vi "DMM Measurement Loop.vi"(3 "error in":errorcluster, 4 "DMM Control References Array":T1, 5 "DMM Semaphore":T2) -> (0 "error out":errorcluster)   [LabVIEW 2020]
uses:
  Typedefs/DMM Control Variable References.ctl
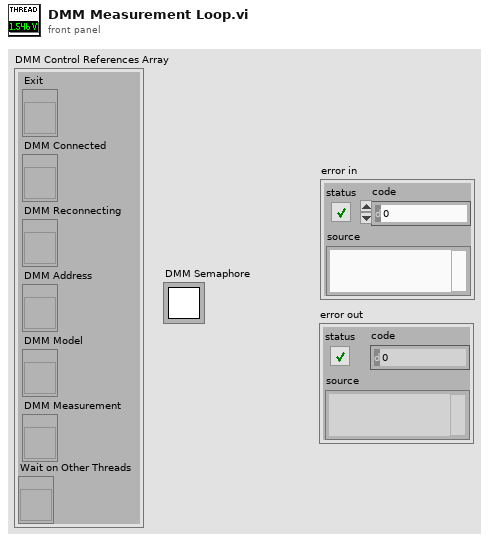
[diagram p1: front panel]
types:
  T1 = typedef "DMM Control Variable References.ctl" = cluster{"Exit":refnum<vi>, "DMM Connected":refnum<vi>, "DMM Reconnecting":refnum<vi>, "DMM Address":refnum<vi>, "DMM Model":refnum<vi>, "DMM Measurement":refnum<vi>, "Wait on Other Threads":refnum<vi>}
  T2 = typedef "Semaphore RefNum" = refnum<k1>
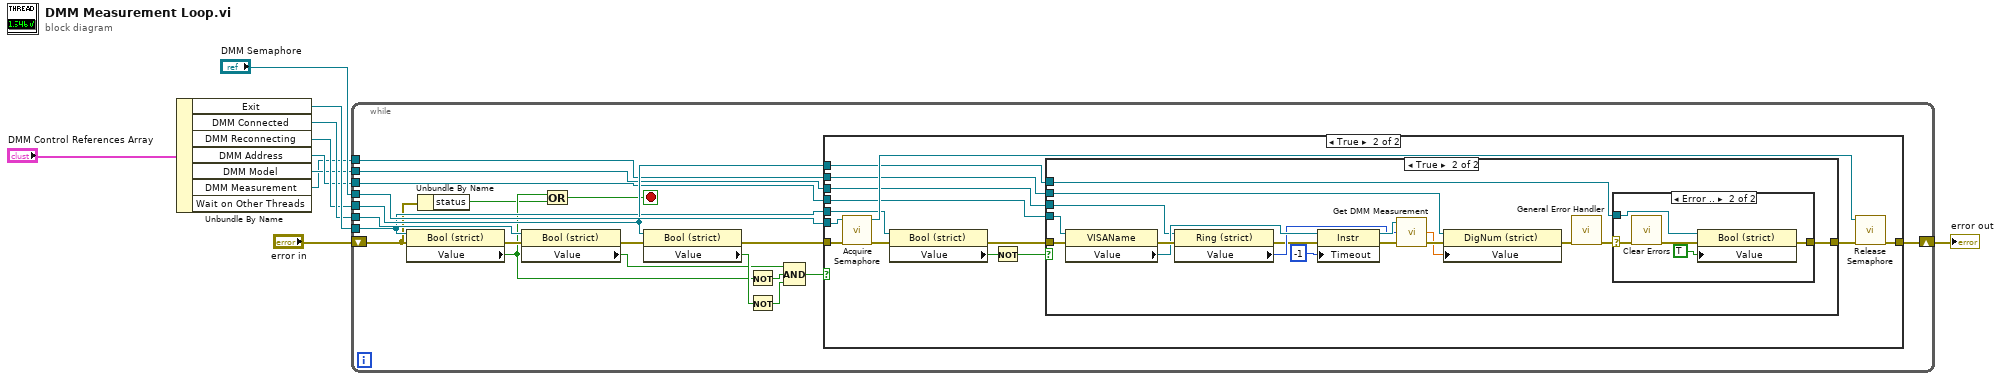
[diagram p0: block diagram]
diagram:
  n1 = Unbundle By Name("DMM Control References Array") -> ("Exit"=w8:refnum<vi>, "DMM Connected"=w7:refnum<vi>, "DMM Reconnecting"=w6:refnum<vi>, "DMM Address"=w5:refnum<vi>, "DMM Model"=w4:refnum<vi>, "DMM Measurement"=w3:refnum<vi>)  [unwired: 1 out]
  n2 = while {
    tunnel: "DMM Semaphore" -> [w30]
    tunnel: w8 -> [w16]
    tunnel: w7 -> [w26]
    tunnel: w6 -> [w20]
    tunnel: w5 -> [w19]
    tunnel: w4 -> [w18]
    tunnel: w3 -> [w17]
    shift-right: [w15] -> w1
    shift-left: "error in" -> [w14]
    stop <- w11 stop-if-true
    n3 = property class="Bool (strict)"(reference=w16, error in=w14) -> (error out=w24:errorcluster, "Value"=w13:bool)  [unwired: 1 out]
    n4 = Unbundle By Name(w14) -> ("status"=w12:bool)
    n5 = property class="Bool (strict)"(reference=w26, error in=w24) -> (error out=w23:errorcluster, "Value"=w21:bool)  [unwired: 1 out]
    n6 = Or(x=w13, y=w12) -> (x .or. y?=w11:bool)
    n7 = property class="Bool (strict)"(reference=w20, error in=w23) -> (error out=w22:errorcluster, "Value"=w25:bool)  [unwired: 1 out]
    n8 = Not(x=w13) -> (.not. x?=w29:bool)
    n9 = Not(x=w25) -> (.not. x?=w28:bool)
    n10 = Compound Arithmetic op=AND(w21, w29, w28) -> (w27:bool)
    n11 = case shown="True" w27 {
      tunnel: w30 -> [_ w45]
      tunnel: w22 -> [w31 w41]
      tunnel: w20 -> [_ w40]
      tunnel: w19 -> [_ w39]
      tunnel: w18 -> [_ w38]
      tunnel: w17 -> [_ w37]
      tunnel: w16 -> [_ w35]
      tunnel: [w31 w32] -> w15
      frame False {
      }
      frame True {
        n12 = call <vilib>:"Acquire Semaphore.vi"("error in (no error)"=w41, "semaphore"=w45) -> ("error out"=w36:errorcluster, "semaphore out"=w43:T2)  [unwired: 3 in, 1 out]
        n13 = property class="Bool (strict)"(reference=w35, error in=w36) -> (error out=w33:errorcluster, "Value"=w34:bool)  [unwired: 1 out]
        n14 = Not(x=w34) -> (.not. x?=w42:bool)
        n15 = case shown="True" w42 {
          tunnel: w33 -> [w46 w57]
          tunnel: [w46 w62] -> w44
          tunnel: w40 -> [_ w58]
          tunnel: w39 -> [_ w55]
          tunnel: w38 -> [_ w53]
          tunnel: w37 -> [_ w50]
          frame False {
          }
          frame True {
            n16 = property class="VISAName"(reference=w55, error in=w57) -> (error out=w56:errorcluster, "Value"=w54:refnum<visa-resource-name>)  [unwired: 1 out]
            n17 = property class="Ring (strict)"(reference=w53, error in=w56) -> (error out=w51:errorcluster, "Value"=w52:u16)  [unwired: 1 out]
            n18 = property class="Instr"(reference=w54, error in=w51, "Timeout"=-1) -> (reference out=w60:refnum<visa-resource-name>, error out=w59:errorcluster)
            n19 = call "Get DMM Measurement.vi"("error in"=w59, "DMM Model"=w52, "DMM Address"=w60) -> ("error out"=w49:errorcluster, "Measurement"=w47:dbl)  [unwired: 1 out]
            n20 = property class="DigNum (strict)"(reference=w50, error in=w49, "Value"=w47) -> (error out=w48:errorcluster)  [unwired: 1 out]
            n21 = call <vilib>:"General Error Handler.vi"("error in (no error)"=w48) -> ("error out"=w63:errorcluster)  [unwired: 10 in, 4 out]
            n22 = case shown="Error .." w63 {
              selector: w63 -> [w64 w69]
              tunnel: [w64 w65] -> w62
              tunnel: w58 -> [_ w68]
              frame No Error {
              }
              frame Error {
                n23 = call <vilib>:"Clear Errors.vi"("error in (no error)"=w69) -> ("error out"=w66:errorcluster)  [unwired: 5 in, 1 out]
                n24 = property class="Bool (strict)"(reference=w68, error in=w66, "Value"=TRUE) -> (error out=w65:errorcluster)  [unwired: 1 out]
              }
            }
          }
        }
        n25 = call <vilib>:"Release Semaphore.vi"("error in (no error)"=w44, "semaphore"=w43) -> ("error out"=w32:errorcluster)  [unwired: 4 in, 1 out]
      }
    }
  }
  "error out" <- w1
